vi "Load Custom Device.vi"(8 "error in":errorcluster, 10 "Custom Device Name":string, 11 "Path":path) -> (0 "error out":errorcluster, 3 "Custom Device out":refnum<class "Custom Device.lvclass">)   [LabVIEW 2027, in "Custom Device Interfaces.lvlib" / "Custom Device Utility.lvclass"]
uses:
  Custom Device Utility.lvclass
  CustomDevice/Custom Device.lvclass
  <vilib>/Utility/LVLibp/NI_PackedLibraryUtility.lvlib
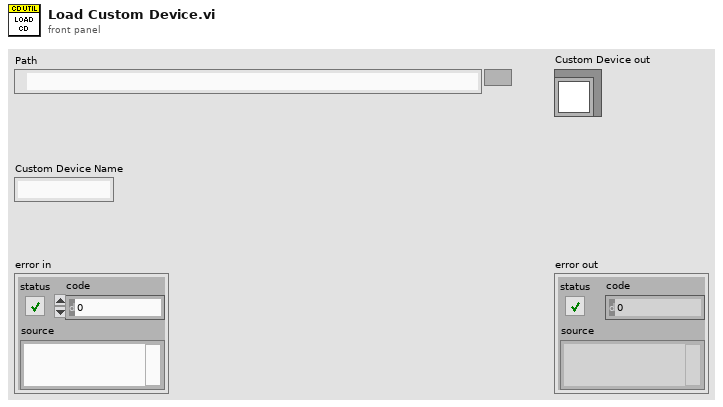
[diagram p1: front panel]
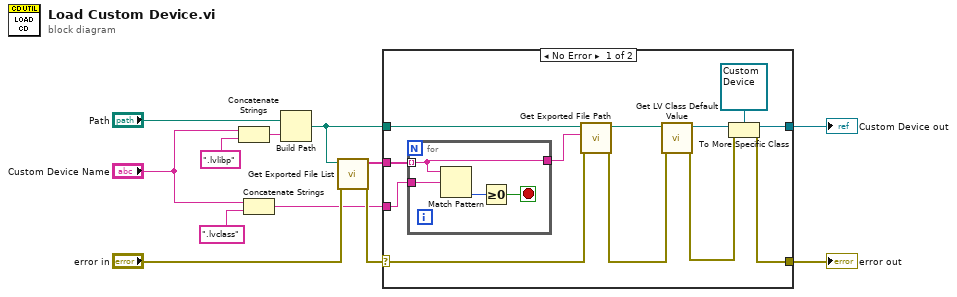
[diagram p0: block diagram]
diagram:
  n1 = Concatenate Strings("Custom Device Name", ".lvlibp") -> (w8:string)
  n2 = Concatenate Strings("Custom Device Name", ".lvclass") -> (w5:string)
  n3 = Build Path(base path="Path", name or relative path=w8) -> (appended path=w4:path)
  n4 = call <vilib>:"Get Exported File List.vi"("error in (no error)"="error in", "packed library path"=w4) -> ("error out"=w11:errorcluster, "qualified names"=w6:string[])  [unwired: 7 in, 1 out]
  n5 = case shown="No Error" w11 {
    selector: w11 -> [w24 w29]
    tunnel: w6 -> [w22 _]
    tunnel: w5 -> [w21 _]
    tunnel: w4 -> [w20 _]
    tunnel: [w18 _] -> w2
    tunnel: [w23 w29] -> w10
    frame No Error {
      n6 = for {
        tunnel: w22 -> [w25] mode=indexing
        tunnel: w21 -> [w28]
        tunnel: [w25] -> w19
        stop <- w26 stop-if-true
        n7 = Match Pattern(string=w25, regular expression=w28) -> (offset past match=w27:i32)  [unwired: 1 in, 3 out]
        n8 = Greater Or Equal To 0?(x=w27) -> (x >= 0?=w26:bool)
      }
      n9 = call <vilib>:"Get Exported File Path.vi"("error in (no error)"=w24, "qualified name"=w19, "packed library path"=w20) -> ("error out"=w17:errorcluster, "path"=w15:path)  [unwired: 7 in]
      n10 = call <vilib>:"Get LV Class Default Value.vi"("error in (no error)"=w17, "class path"=w15) -> ("error out"=w16:errorcluster, "object"=w13:refnum<class>)  [unwired: 8 in]
      n11 = To More Specific Class(target class=refnum<class "Custom Device.lvclass"> refnum, reference=w13, error in=w16) -> (specific class reference=w18:refnum<class "Custom Device.lvclass">, error out=w23:errorcluster)
    }
    frame Error {
    }
  }
  "Custom Device out" <- w2
  "error out" <- w10
